vi "Lines LoadArrayOfSessions.vi"(7 "Annotation Separator(#)":string="#", 8 "error in (no error)":errorcluster, 10 "Session Name":string, 11 "Lines":string[](array[string])) -> (0 "error out":errorcluster, 1 "Matched Sessions":string[](array[string]), 2 "String Config Group":cluster{"Key":string, "Value":string}[](array[cluster]), 3 "Config Text List out":string[](array[string]))   [LabVIEW 2017, in "ini_configuration.lvlib"]
doc: "Loads the session named Session Name from Lines and returns it both as a list of lines and as an array of key-value pairs, with the annotation lines removed."
uses:
  ini_configuration.lvlib
  _openG/_reuse_openG.lvlib
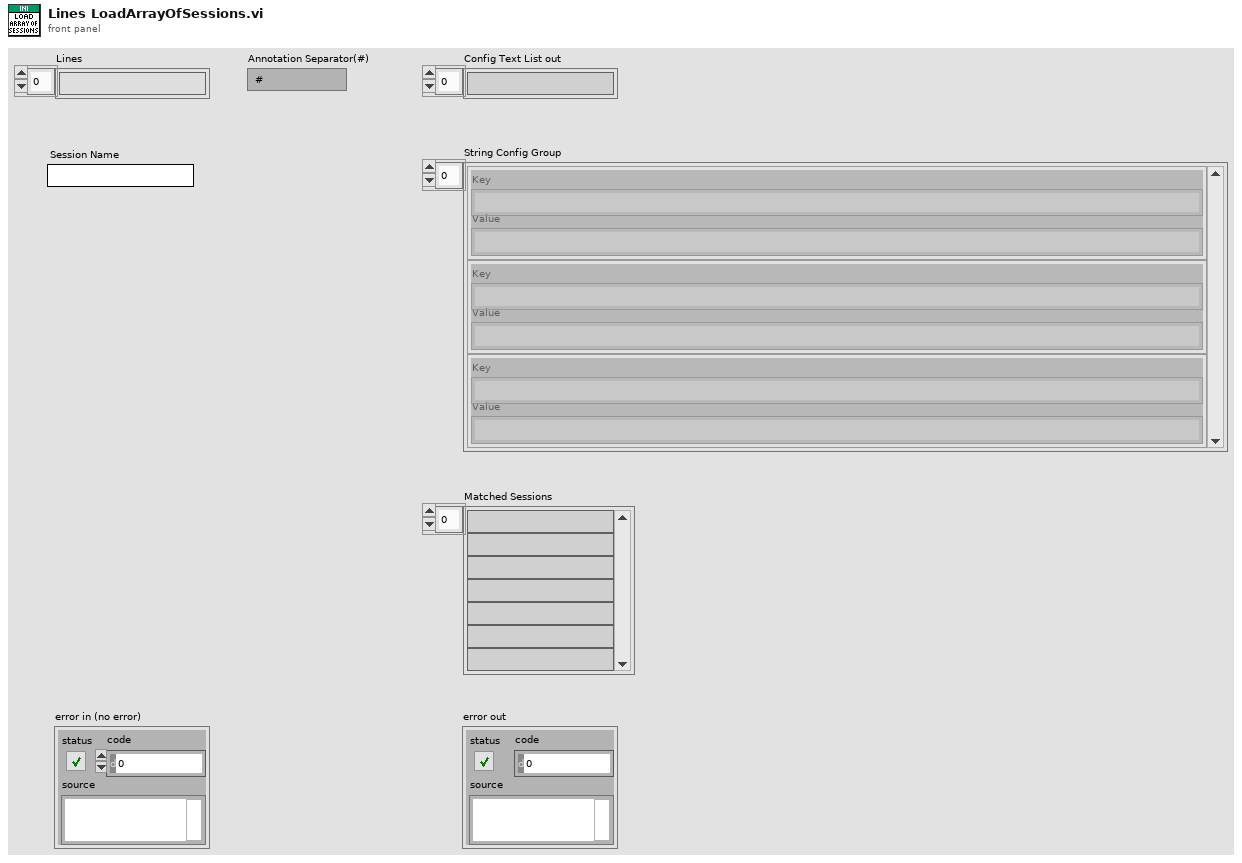
[diagram p1: front panel]
types:
  T1 = cluster{"name":string, "trimmed string":string}[]
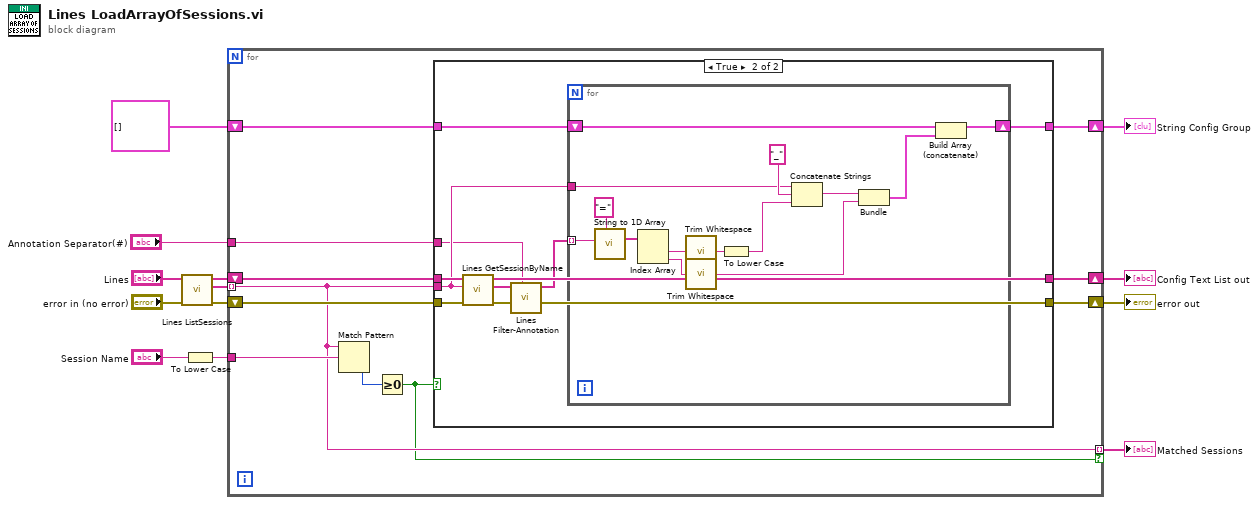
[diagram p0: block diagram]
diagram:
  n1 = call "Lines ListSessions.vi"("error in (no error)"="error in (no error)", "Config Text List"="Lines") -> ("error out"=w7:errorcluster, "Sessions"=w10:string[], "Config Text List out"=w8:string[])  [unwired: 7 in]
  n2 = To Lower Case(string="Session Name") -> (all lower case string=w13:string)
  n3 = for {
    shift-right: [w22] -> w9
    shift-left: w8 -> [w23]
    tunnel: w10 -> [w16] mode=indexing
    shift-right: [w20] -> w11
    shift-left: w7 -> [w24]
    tunnel: w13 -> [w19]
    shift-right: [w18] -> w3
    shift-left: cluster{"name":string, "cfg":string}[] [] ("String Config Group") -> [w17]
    tunnel: [w16] -> w2 mode=indexing if=w15
    tunnel: "Annotation Separator(#)" -> [w14]
    n4 = Match Pattern(string=w16, regular expression=w19) -> (offset past match=w21:i32)  [unwired: 1 in, 3 out]
    n5 = Greater Or Equal To 0?(x=w21) -> (x >= 0?=w15:bool)
    n6 = case shown="True" w15 {
      tunnel: w24 -> [w26 w37]
      tunnel: w23 -> [w27 w35]
      tunnel: [w27 w34] -> w22
      tunnel: w16 -> [_ w32]
      tunnel: [w26 w31] -> w20
      tunnel: [w25 w30] -> w18
      tunnel: w17 -> [w25 w29]
      tunnel: w14 -> [_ w28]
      frame False {
      }
      frame True {
        n7 = call "Lines GetSessionByName.vi"("error in (no error)"=w37, "[] Session Name"=w32, "Config Text List"=w35) -> ("error out"=w38:errorcluster, "Session"=w36:string[], "Config Text List out"=w34:string[])  [unwired: 6 in]
        n8 = call "Lines Filter-Annotation.vi"("Annotation Separator(#)"=w28, "error in (no error)"=w38, "Lines"=w36) -> ("error out"=w31:errorcluster, "Config Text List"=w33:string[])  [unwired: 7 in]
        n9 = for {
          tunnel: w33 -> [w48] mode=indexing
          tunnel: w32 -> [w46]
          shift-right: [w43] -> w30
          shift-left: w29 -> [w44]
          n10 = call "String to 1D Array.vi"("delimiter (Tab)"="=", "string"=w48) -> ("Array of Strings"=w50:string[])  [unwired: 9 in]
          n11 = Index Array(array=w50) -> (element #1=w51:string, element #2=w52:string)  [unwired: 2 in]
          n12 = call <vilib>:"Trim Whitespace.vi"("string"=w51) -> ("trimmed string"=w45:string)  [unwired: 1 in]
          n13 = call <vilib>:"Trim Whitespace.vi"("string"=w52) -> ("trimmed string"=w41:string)  [unwired: 1 in]
          n14 = To Lower Case(string=w45) -> (all lower case string=w39:string)
          n15 = Concatenate Strings(w46, "_" ("delimiter (Tab)"), w39) -> (w42:string)
          n16 = Bundle(w42, "trimmed string"=w41) -> (w40:cluster{string, "trimmed string":string})  [unwired: 1 in]
          n17 = Build Array (concatenate)(w44, w40) -> (w43:T1)
        }
      }
    }
  }
  "error out" <- w11
  "Config Text List out" <- w9
  "String Config Group" <- w3
  "Matched Sessions" <- w2
